vi "SearchACKs(byID).vi"(8 "error in (no error)":errorcluster, 10 "Packet Identifier":u16 format="%016b", 11 "Session in":refnum<class "Session.lvclass">) -> (0 "error out":errorcluster, 1 "found?":bool, 2 "Pending ACK":T1 {"Packet Identifier" format="%016b"}, 3 "Session out":refnum<class "Session.lvclass">)   [LabVIEW 2013, in "MQTT Server.lvlib" / "Session.lvclass"]
uses:
  Session.lvclass
  Pending ACKs -- cluster.ctl
  Control Packets/ControlPacket/ControlPacket.lvclass
  Session.lvclass/Session.ctl
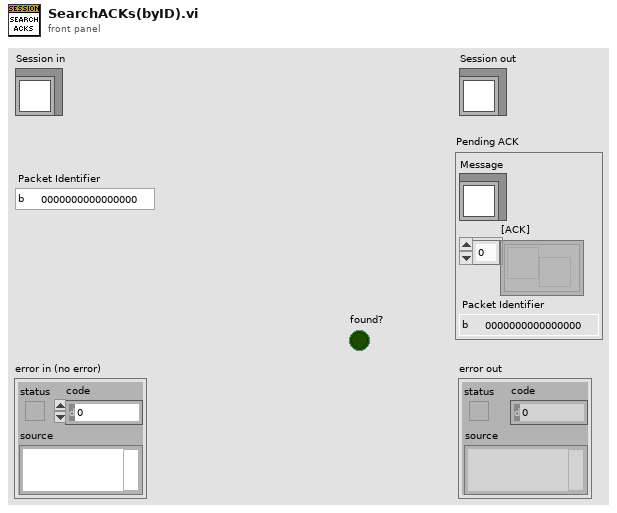
[diagram p1: front panel]
types:
  T1 = typedef "MQTT Server.lvlib/Session.lvclass/Pending ACKs -- cluster.ctl" = cluster{"Message":refnum<class "ControlPacket.lvclass">, "[ACK]":refnum<notifier>[], "Packet Identifier":u16}
  T2 = typedef "MQTT Server.lvlib/Session.lvclass/Session State -- cluster.ctl" = cluster{"CleanSession":bool, "Client ID":string, "Subscriptions":T3[], "Pending Transmissions":T5[], "Pending ACKs":T1[]}
  T3 = typedef "SUBSCRIBE.lvclass/Topic Subscription -- cluster.ctl" = cluster{"Topic Filter":string, "QoS":T4}
  T4 = typedef "ControlPacket.lvclass/QualityOfService -- enum.ctl" = enum16{"0 (At Most Once)", "1 (At Least Once)", "2 (Exactly Once)"}
  T5 = typedef "ControlPacket.lvclass/Pending Transmission -- cluster.ctl" = cluster{"Message":refnum<class "ControlPacket.lvclass">, "QoS":T4, "Tx-Rx":bool}
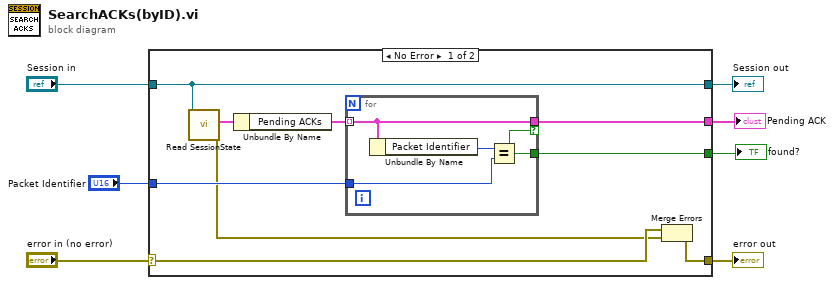
[diagram p0: block diagram]
diagram:
  n1 = case shown="No Error" "error in (no error)" {
    selector: "error in (no error)" -> [w16 w21]
    tunnel: [w15 w21] -> w6
    tunnel: [w14 w22] -> w4
    tunnel: "Session in" -> [w14 w22]
    tunnel: "Packet Identifier" -> [w11 _]
    tunnel: [w10 _] -> w2
    tunnel: [w9 _] -> w1
    frame No Error {
      n2 = call "Read SessionState.vi"("Session in"=w14) -> ("error out"=w8:errorcluster, "Session State"=w13:T2)  [unwired: 8 in, 1 out]
      n3 = Unbundle By Name(w13) -> ("Pending ACKs"=w12:T1[])
      n4 = for {
        tunnel: w12 -> [w20] mode=indexing
        tunnel: [w20] -> w9 if=w17
        tunnel: w11 -> [w18]
        tunnel: [w17] -> w10
        n5 = Unbundle By Name(w20) -> ("Packet Identifier"=w19:u16)
        n6 = Equal?(x=w19, y=w18) -> (x = y?=w17:bool)
      }
      n7 = Merge Errors(w16, w8) -> (w15:errorcluster)
    }
    frame Error {
    }
  }
  "error out" <- w6
  "Session out" <- w4
  "Pending ACK" <- w1
  "found?" <- w2
